vi "CreateWO-VerifyWordDocCreated.vi"(8 "error in (no error)":errorcluster, 10 "Path for Saving the file":path, 11 "Automation Refnum in":refnum<k7>) -> (0 "error out":errorcluster, 2 "Word Doc Not Created":bool, 3 "Automation Refnum out":refnum<k7>)   [LabVIEW 2013, in "ERP-CreateWorkOrder.lvclass"]
uses:
  ERP-CreateWorkOrder.lvclass
  <userlib>/_OpenG.lib/file/file.llb/Valid Path - Traditional__ogtk.vi
  <vilib>/Utility/error.llb/Error Cluster From Error Code.vi
  <vilib>/ErrorRing/Error Ring.xnode
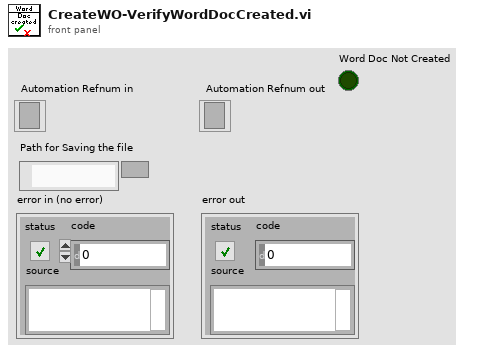
[diagram p1: front panel]
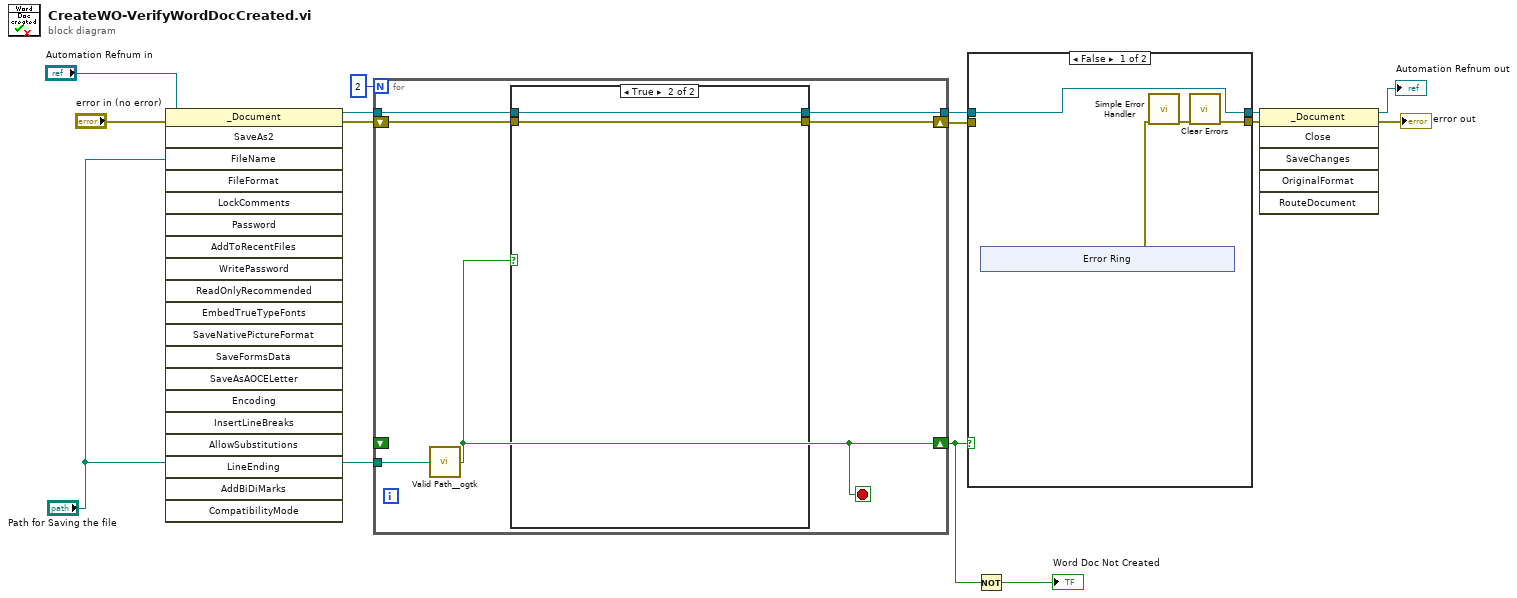
[diagram p0: block diagram]
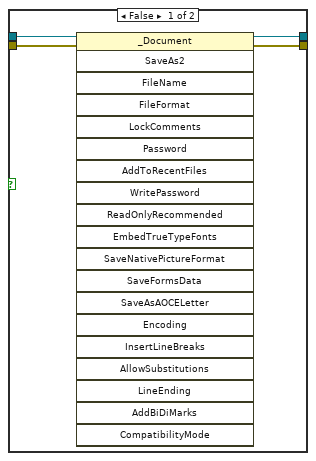
[diagram p3: hidden frame]
diagram:
  n1 = invoke class="_Document" method="SaveAs2"(reference="Automation Refnum in", error in="error in (no error)", "FileName"="Path for Saving the file") -> (reference out=w10:refnum<k7>, error out=w11:errorcluster)  [unwired: 17 in, 18 out]
  n2 = for {
    N: 2 -> [_]
    tunnel: "Path for Saving the file" -> [w20]
    shift-right: [w17] -> w2
    shift-left: _ -> [_]
    tunnel: w10 -> [w18]
    shift-right: [w16] -> w8
    shift-left: w11 -> [w19]
    tunnel: [w15] -> w7
    stop <- w17 stop-if-true
    n3 = call-poly <userlib>:"Valid Path__ogtk.vi"("path"=w20) -> ("valid"=w17:bool)
    n4 = case shown="True" w17 {
      tunnel: w19 -> [w24 w26]
      tunnel: w18 -> [w23 w25]
      tunnel: [w22 w26] -> w16
      tunnel: [w21 w25] -> w15
      frame False {
        n5 = invoke class="_Document" method="SaveAs2"(reference=w23, error in=w24) -> (reference out=w21:refnum<k7>, error out=w22:errorcluster)  [unwired: 18 in, 18 out]
      }
      frame True {
      }
    }
  }
  n6 = case shown="False" w2 {
    tunnel: w8 -> [_ w37]
    tunnel: w7 -> [w27 w36]
    tunnel: [w28 w37] -> w6
    tunnel: [w27 w36] -> w5
    frame False {
      n7 = xnode "Error Ring"() -> ("error out"=w30:errorcluster)
      n8 = call <vilib>:"Simple Error Handler.vi"("error in (no error)"=w30) -> ("error out"=w29:errorcluster)  [unwired: 4 in, 4 out]
      n9 = call <vilib>:"Clear Errors.vi"("error in (no error)"=w29) -> ("error out"=w28:errorcluster)  [unwired: 6 in]
    }
    frame True {
    }
  }
  n10 = Not(x=w2) -> (.not. x?=→"Word Doc Not Created":bool)
  n11 = invoke class="_Document" method="Close"(reference=w5, error in=w6) -> (reference out=→"Automation Refnum out":refnum<k7>, error out=→"error out":errorcluster)  [unwired: 4 in, 4 out]
